vi "KundtsTube.vi"() -> ()   [LabVIEW 2015]
uses:
  <vilib>/imath/engines/lvmath2/RunTimeEngine/Managers/WorkSpace/UID Generator.vi
  <vilib>/imath/engines/lvmath2/RunTimeEngine/RunTimeType/NIMS_RunTimeType_From StrictType (excl LVString).vi
  <instcachedir>/0/NIMS_RunTimeType_From StrictType (excl LVString)_EB1C38A9BC5048DA9ABDA8F781E54D21.lvgen/NIMS_RunTimeType_From StrictType (excl LVString)_EB1C38A9BC5048DA9ABDA8F781E54D21_000.vi
  <vilib>/imath/engines/lvmath2/RunTimeEngine/LocalVariableDefStatement/MC_LocalVariableDefStatement_Display.vi
  <vilib>/imath/engines/lvmath2/RunTimeEngine/Managers/SymbolTable/Clear UID.vi
  <vilib>/imath/engines/lvmath2/RunTimeEngine/NodeEndStatement/NIMS_NodeEndStatement_Output.vi
  <instcachedir>/0/NIMS_NodeEndStatement_Output_53EC0D466D134D7ABD903AC30B43404B.lvgen/NIMS_NodeEndStatement_Output_53EC0D466D134D7ABD903AC30B43404B_009.vi
  <vilib>/imath/engines/lvmath2/RunTimeEngine/ErrorHandling/NIMS_Finalize Error.vi
  <vilib>/Utility/file.llb/Write Delimited Spreadsheet (DBL).vi
  <vilib>/imath/engines/lvmath2/RunTimeEngine/Managers/SymbolTable/NIMS_WorkSpace.lvlib
panel:
  in  "Tab Control":enum32{"Single Frequency", "Sweep"}(tab)=enum."Sweep"
  in  "Frequency 2":dbl=10.1 caption="Frequency"
  in  "Dwell Time (s)":dbl=0.5
  out "Gain vs Frequency":cluster{"Output Array":dbl[], dbl[]}(graph)={"Output Array"=[10.0, 94.0, 178.0, 262.0, 346.0, 430.0, 514.0, 598.0, 682.0, 766.0, 849.0, 933.0, 1017.0, 1101.0, 1185.0, 1269.0, 1353.0, 1437.0, 1521.0, 1605.0, 1689.0, 1773.0, 1857.0, 1941.0, 2025.0, 2109.0, 2193.0, 2277.0, 2361.0, 2445.0, 2528.0, 2612.0, 2696.0, 2780.0, 2864.0, 2948.0, 3032.0, 3116.0, 3200.0, 3284.0, 3368.0, 3452.0, 3536.0, 3620.0, 3704.0, 3788.0, 3872.0, 3956.0, 4040.0, 4124.0, 4207.0, 4291.0, 4375.0, 4459.0, 4543.0, 4627.0, 4711.0, 4795.0, 4879.0, 4963.0, 5047.0, 5131.0, 5215.0, 5299.0, 5383.0, 5467.0, 5551.0, 5635.0, 5719.0, 5803.0, 5886.0, 5970.0, 6054.0, 6138.0, 6222.0, 6306.0, 6390.0, 6474.0, 6558.0, 6642.0, 6726.0, 6810.0, 6894.0, 6978.0, 7062.0, 7146.0, 7230.0, 7314.0, 7398.0, 7482.0, 7565.0, 7649.0, 7733.0, 7817.0, 7901.0, 7985.0, 8069.0, 8153.0, 8237.0, 8321.0, 8405.0, 8489.0, 8573.0, 8657.0, 8741.0, 8825.0, 8909.0, 8993.0, 9077.0, 9161.0, 9244.0, 9328.0, 9412.0, 9496.0, 9580.0, 9664.0, 9748.0, 9832.0, 9916.0, 10000.0], [-135.47380641049241, -134.395560313578, -135.31931377816244, -104.67314630566749, -70.52224777984337, -77.95730123384658, -62.76312624369845, -69.12715538357209, -61.2250530781428, -69.41486490773038, -66.03242754906071, -71.17706349802742, -73.1812849189445, -74.74562256229484, -80.12023457252104, -76.42737109092013, -85.78275073892618, -77.52531553543587, -90.4619209747234, -77.86043590724384, -93.84548215650368, -76.3212326371636, -97.52628172990293, -74.54251085502531, -99.94203316131751, -70.5287761085898, -101.75425193469906, -61.709653445958565, -105.11070694251403, -56.29502390080326, -105.80028781985686, -68.7641465070975, -106.28045505849173, -79.08028001683597, -107.0809577999689, -88.41580870527322, -107.54640289844396, -94.784838592432, -107.17669144724229, -100.1361356834849, -106.47699534879737, -104.08611352898953, -104.73012276801683, -93.84871516028012, -100.90959121943355, -109.04020470839936, -100.82860451895661, -110.20257184067654, -97.67950847435044, -102.29962283132252, -92.90916036060766, -110.6606185611997, -88.76848609780082, -110.46022290461107, -82.49995461535372, -110.93094342686543, -73.32621080937199, -109.45755620184522, -70.4607321298734, -109.60643716320874, -79.43358474464975, -106.93826146885287, -87.03092007940376, -105.66498279259206, -93.97336876614628, -102.88073132662024, -99.29058869665428, -100.15010380877476, -103.37880650172109, -95.58904539965408, -106.0551426484403, -89.53203604544571, -108.83594415683098, -83.42402882357402, -111.32670382754775, -77.1035716782684, -112.34112275384369, -81.74419354287615, -113.98321924205015, -91.1597915351306, -114.444194727013, -98.61386505802848, -115.3559770108955, -104.61739887029084, -116.41515835012086, -109.31220592948138, -115.34399736679734, -109.89315177349197, -114.31166606829754, -115.45825408835623, -111.64787684539739, -118.10802594522806, -110.16367170912642, -119.63073846699386, -105.49098106833695, -121.37681563872147, -98.50499965514598, -121.7219469667147, -93.49565867165671, -122.44787885958897, -100.65064592369816, -122.83369211866535, -109.19595496580692, -123.07221033094638, -115.5822064532059, -123.27527921467836, -119.95615560661824, -121.77966922462832, -122.430808406013, -119.65632878908751, -124.44500166337085, -118.23187550925846, -126.00067881286765, -115.68550395652666, -126.39026298830542, -110.30540327012979, -127.33914739175552, -105.79881121084014, -128.29764678089245, -110.52049996377774, -127.47251571807011, -119.08054002496303]}
  out "RMS output":dbl=0.005190735792344873 format="%0.2f"
  in  "Number of Points":dbl=120.0
  in  "stop":bool
  out "Waveform":dynamicdata(graph)=[{"t0"=timestamp(3530217010.2415156 s since 1904-01-01), "dt"=9.999999999999972e-06, "Y"=array[100000 elements], "attributes"=variant("NI_ChannelName"=variant(string "Voltage"), "NI_UnitDescription"=variant(string "Volts"))}]
  in  "Sampling Rate":dbl=100000.0
  in  "number of samples":i32=100000
  out "error out":errorcluster={"status"=FALSE, "code"=200015, "source"="SignalGenerator.vi:Instance:8:560001"}
  in  "Amplitude":dbl=2.0
  out "Frequency":dbl
  in  "Spacing":u16(ring) items=["Linear", "Logarithmic"]
  in  "Maximim":dbl=10000.0
  in  "Minimum":dbl=10.0
  # "Sweep from min to max frequency\npausing by the dwell time between \neach iteration"
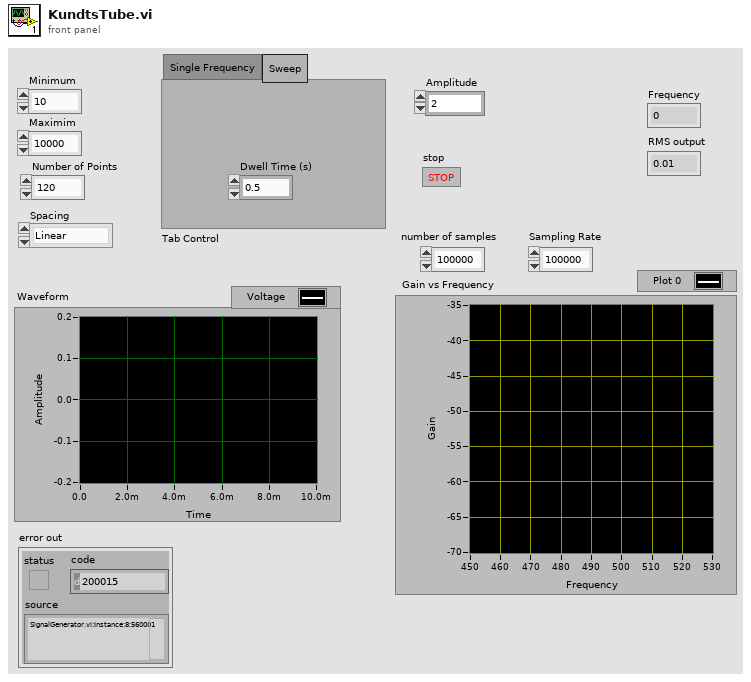
[diagram p1: front panel]
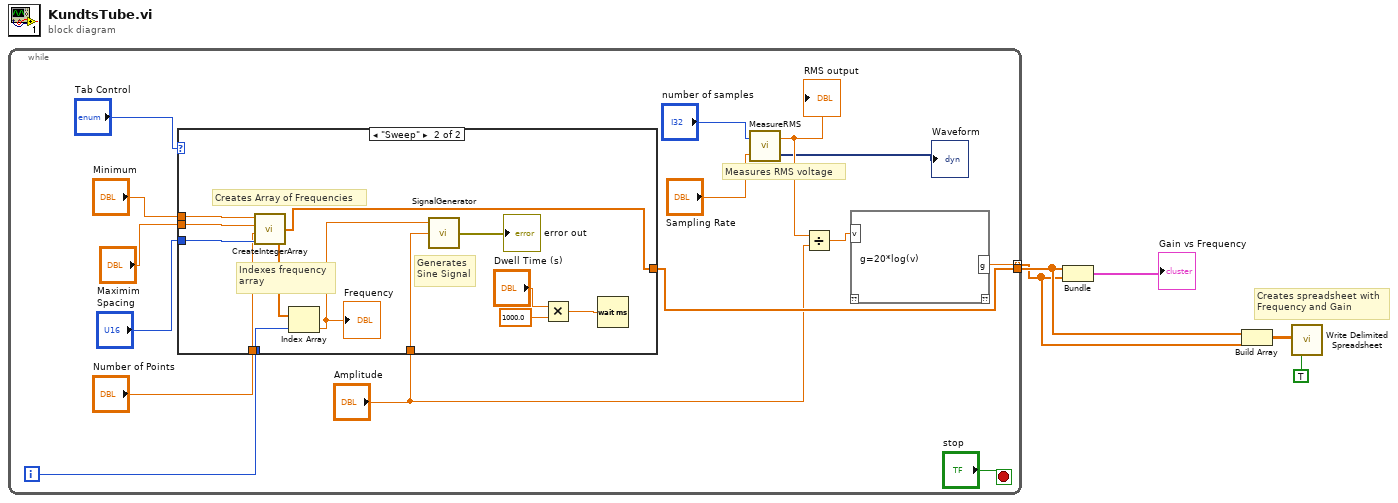
[diagram p0: block diagram]
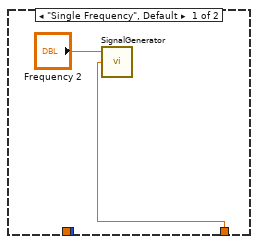
[diagram p2: hidden frame]
diagram:
  # "Creates spreadsheet with\nFrequency and Gain"
  n1 = while {
    tunnel: [w10] -> w2 mode=indexing
    tunnel: [w9] -> w3
    i -> [w20]
    stop <- "stop" stop-if-true
    # "Measures RMS voltage"
    n2 = case shown="\"Sweep\"" "Tab Control" {
      tunnel: w20 -> [_ w71]
      tunnel: "Minimum" -> [_ w68]
      tunnel: "Maximim" -> [_ w67]
      tunnel: "Spacing" -> [_ w66]
      tunnel: "Number of Points" -> [_ w65]
      tunnel: [_ w61] -> w9
      tunnel: "Amplitude" -> [w58 w60]
      frame "Single Frequency", Default {
        n3 = call "SignalGenerator.vi"("Amplitude"=w58, "Frequency"="Frequency 2") -> ()  [unwired: 1 in, 1 out]
      }
      frame "Sweep" {
        # "Indexes frequency\narray"
        # "Generates \nSine Signal"
        # "Creates Array of Frequencies"
        n4 = call "CreateIntegerArray.vi"("Spacing"=w66, "Number of Points"=w65, "Maximim"=w67, "Minimum"=w68) -> ("Output Array"=w61:dbl[])
        n5 = Index Array(array=w61, index=w71) -> (element=w70:dbl)
        "Frequency" <- w70
        n6 = call "SignalGenerator.vi"("Amplitude"=w60, "Frequency"=w70) -> ("error out"=→"error out":errorcluster)  [unwired: 1 in]
        n7 = Multiply(x="Dwell Time (s)", y=1000.0) -> (x*y=w64:dbl)
        n8 = Wait (ms)(milliseconds to wait=w64) -> ()  [unwired: 1 out]
      }
    }
    n9 = call "MeasureRMS.vi"("rate"="Sampling Rate", "number of samples"="number of samples") -> ("data"=→"Waveform":dynamicdata, "AC estimate (Vrms)"=w12:dbl)
    "RMS output" <- w12
    n10 = Divide(x=w12, y="Amplitude") -> (x/y=w11:dbl)
    n11 = mathscript code="g=20*log(v)"("v"=w11) -> ("g"=w10:cdb)  [unwired: 1 in, 1 out]
  }
  n12 = Bundle("Output Array"=w3, w2) -> (→"Gain vs Frequency":cluster{"Output Array":dbl[], cdb[]})  [unwired: 1 in]
  n13 = Build Array(w3, w2) -> (w1:cdb[][])
  n14 = call-poly <vilib>:"Write Delimited Spreadsheet.vi"("2D data"=w1, "transpose? (F)"=TRUE) -> ()  [unwired: 12 in, 2 out]
